vi "Search_Element.vi"() -> ()   [LabVIEW 2024]
panel:
  out "index of element":i32
  in  "1D array":dbl[](array[numeric])
  in  "element":dbl
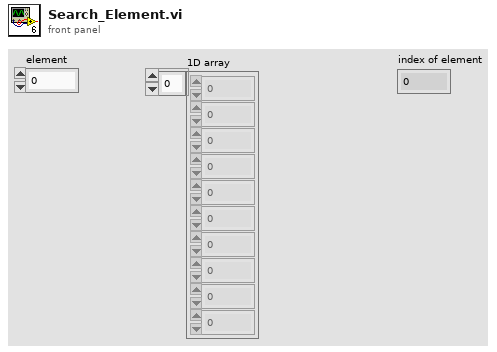
[diagram p1: front panel]
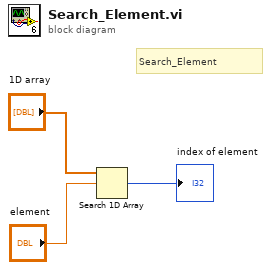
[diagram p0: block diagram]
diagram:
  # "Search_Element"
  n1 = Search 1D Array(1D array="1D array", element="element") -> (index of element=→"index of element":i32)  [unwired: 1 in]
